vi "try.vi"() -> ()   [LabVIEW 2015]
uses:
  <vilib>/addons/_JKI.lib/REST Client/classes/REST Client/REST Client.lvclass
  <vilib>/httpClient/LabVIEWHTTPClient.lvlib
  <vilib>/httpClient/MultipartData.ctl
  <vilib>/addons/_JKI.lib/REST Client/classes/REST Client/HTTP Header.ctl
panel:
  out "error out":errorcluster
  out "Status Code 2":u16
  out "headers":string
  out "body":string
  in  "url":string
  out "error out 3":errorcluster
  in  "Same Params?":bool
  out "Status String":string
  out "Response body posting":string
  out "error out  2":errorcluster
  in  "Post Path":string="/v1/document_revisions/external/0b9ed9ad-4393-4a37-838e-578edaaebe9e"
  in  "Default Headers ([JSON]) 2":T1[](array[typedef])=[{"header"="Content-Type", "value"="application/json"}]
  in  "Base URL Posting":string="https://api.dev.enlil.io/api"
  out "Local Cluster":T2
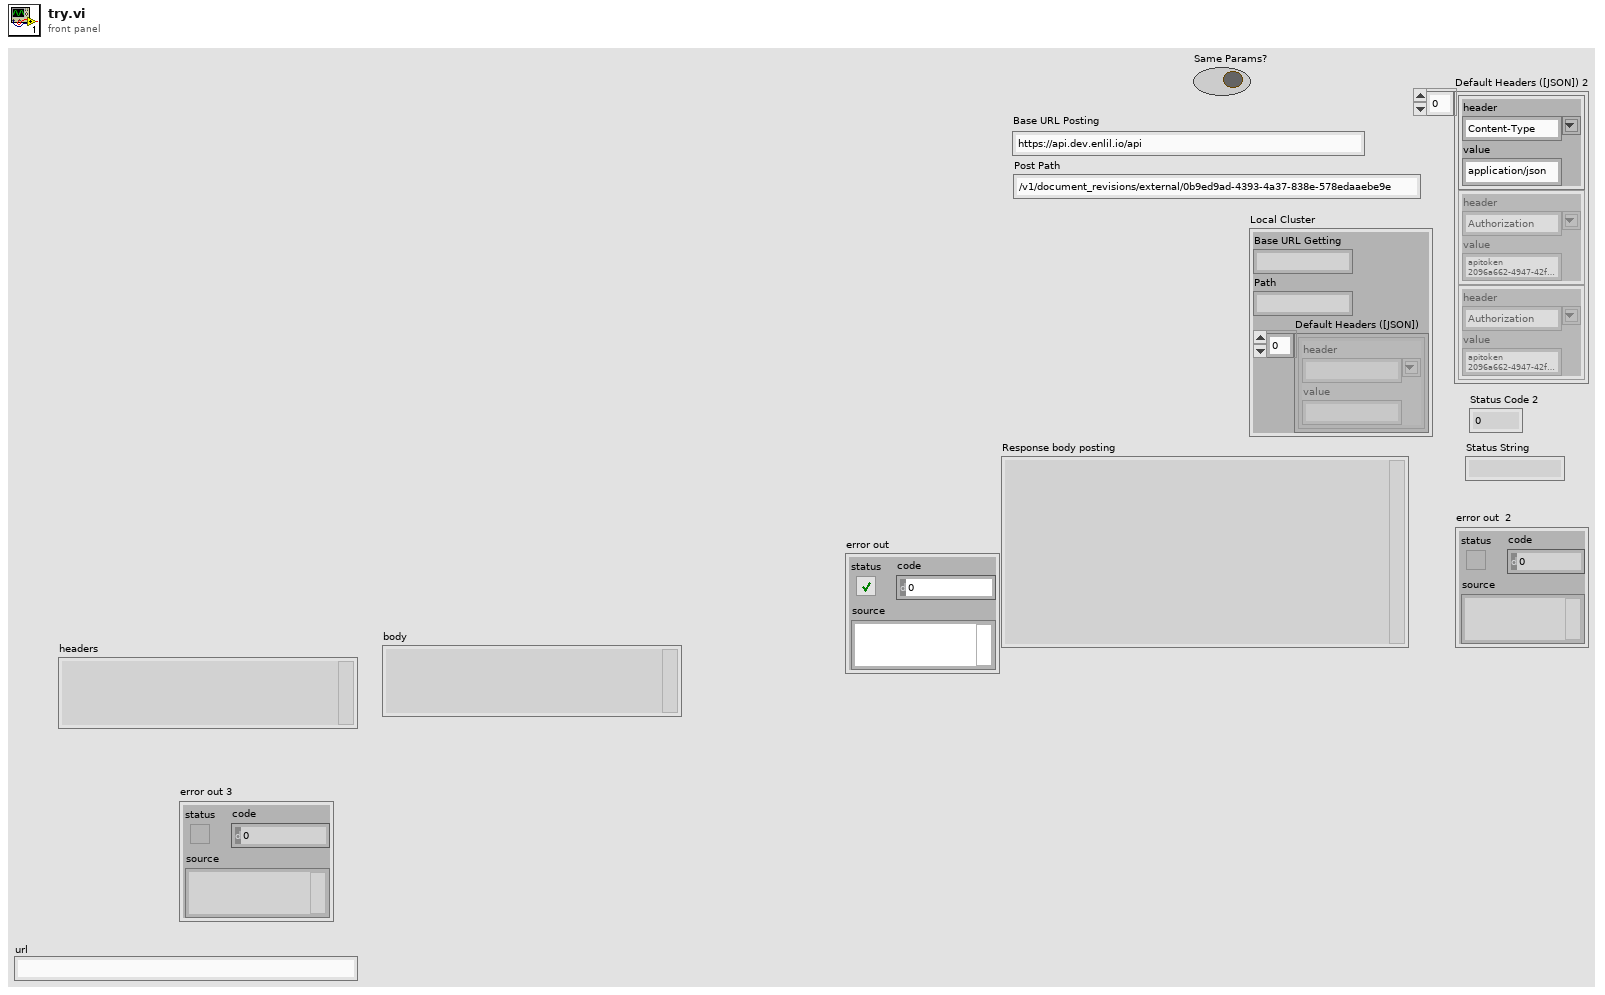
[diagram p1: front panel]
types:
  T1 = typedef "REST Client.lvlib/REST Client.lvclass/HTTP Header.ctl" = cluster{"header":string, "value":string}
  T2 = cluster{"Base URL Getting":string, "Path":string, "Default Headers ([JSON])":T1[]}
  T3 = typedef "LabVIEWHTTPClient.lvlib/MultipartData.ctl" = cluster{"Name":string, "Value":string, "File":path, "Filename":string, "MIME type":string}
  T4 = typedef "LabVIEWHTTPClient.lvlib/ClientHandle.ctl" = refnum<k1>
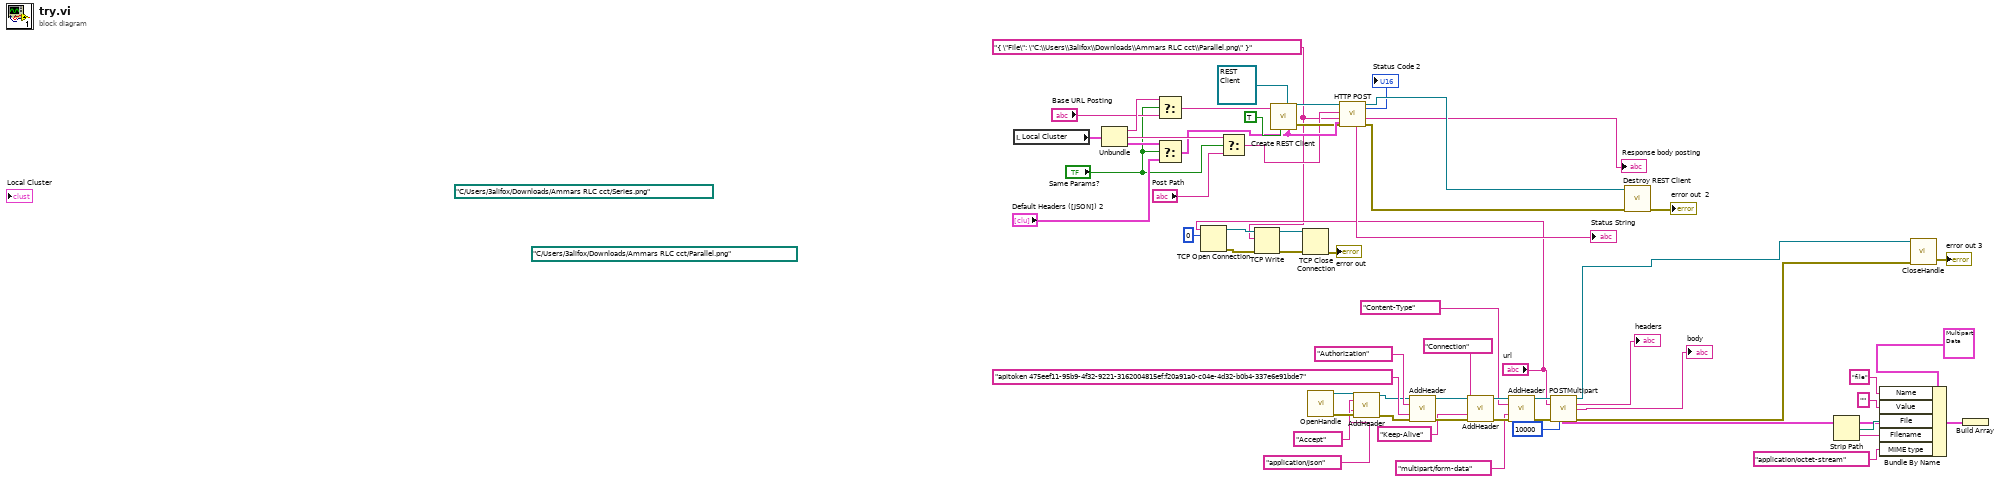
[diagram p0: block diagram]
diagram:
  (unwired) path "C:/Users/3alifox/Downloads/Ammars RLC cct/Series.png" ("Path")
  (unwired) path "C:/Users/3alifox/Downloads/Ammars RLC cct/Parallel.png" ("path to PNG file")
  w5 = "{ \"File\": \"C:\\Users\\3alifox\\Downloads\\Ammars RLC cct\\Parallel.png\" }" ("Request body")
  n1 = local read "Local Cluster"() -> (w58:T2)
  n2 = Unbundle(w58) -> ("Base URL Getting"=w57:string, "Path"=w52:string, "Default Headers ([JSON])"=w54:T1[])
  n3 = Select(t=w57, s="Same Params?", f="Base URL Posting") -> (s? t:f=w55:string)
  n4 = Select(t=w54, s="Same Params?", f="Default Headers ([JSON]) 2") -> (s? t:f=w46:T1[])
  n5 = TCP Open Connection(address="url", remote port or service name=u16 0) -> (connection ID=w8:refnum<k5>, error out=w11:errorcluster)  [unwired: 3 in]
  n6 = Select(t=w52, s="Same Params?", f="Post Path") -> (s? t:f=w43:string)
  n7 = TCP Write(connection ID=w8, data in=w5, error in (no error)=w11) -> (connection ID out=w9:refnum<k5>, error out=w10:errorcluster)  [unwired: 1 in, 1 out]
  n8 = call <vilib>:"Create REST Client.vi"("Default Headers ([JSON])"=w46, "REST Client in"=refnum<class "REST Client.lvclass"> refnum, "Verify Server(true)"=TRUE, "Base URL"=w55) -> ("error out"=w45:errorcluster, "REST Client out"=w47:refnum<class "REST Client.lvclass">)  [unwired: 6 in]
  n9 = TCP Close Connection(connection ID=w9, error in (no error)=w10) -> (error out=→"error out":errorcluster)  [unwired: 1 in, 1 out]
  n10 = call <vilib>:"OpenHandle.vi"() -> ("client handle out"=w15:T4, "error out"=w17:errorcluster)  [unwired: 14 in]
  n11 = call-dynamic "HTTP POST.vi"("request specific headers"=w46, "error in (no error)"=w45, "Request body"=w5, "Path"=w43, "REST Client in"=w47) -> ("error out"=w39:errorcluster, "Response body"=→"Response body posting":string, "REST Client out"=w44:refnum<class "REST Client.lvclass">, "Status String"=→"Status String":string, "Status Code"=→"Status Code 2":u16)  [unwired: 1 in, 1 out]
  n12 = call <vilib>:"AddHeader.vi"("client handle"=w15, "header"="Accept", "value"="application/json", "error in (no error)"=w17) -> ("client handle out"=w14:T4, "error out"=w16:errorcluster)  [unwired: 10 in]
  n13 = call <vilib>:"AddHeader.vi"("client handle"=w14, "header"="Authorization", "value"="apitoken 475eef11-95b9-4f32-9221-3162004815ef:f20a91a0-c04e-4d32-b0b4-337e6e91bde7", "error in (no error)"=w16) -> ("client handle out"=w26:T4, "error out"=w27:errorcluster)  [unwired: 10 in]
  n14 = call <vilib>:"AddHeader.vi"("client handle"=w26, "header"="Connection", "value"="Keep-Alive", "error in (no error)"=w27) -> ("client handle out"=w22:T4, "error out"=w23:errorcluster)  [unwired: 10 in]
  n15 = call <vilib>:"AddHeader.vi"("client handle"=w22, "header"="Content-Type", "value"="multipart/form-data", "error in (no error)"=w23) -> ("client handle out"=w19:T4, "error out"=w18:errorcluster)  [unwired: 10 in]
  n16 = call-dynamic "Destroy REST Client.vi"("error in (no error)"=w39, "REST Client in"=w44) -> ("error out"=→"error out  2":errorcluster)  [unwired: 9 in]
  n17 = Strip Path() -> (path=w3:path, name=w35:string)  [unwired: 1 out]
  n18 = Bundle By Name(cluster=T3 {"Name"="", "Value"="", "File"=path "", "Filename"="", "MIME type"="application/octet-stream"} ("Element"), "Name"="file", "Value"="", "File"=w3, "Filename"=w35, "MIME type"="application/octet-stream") -> (w37:T3)
  n19 = Build Array(w37) -> (w1:T3[])
  n20 = call <vilib>:"POSTMultipart.vi"("client handle"=w19, "url"="url", "data"=w1, "error in (no error)"=w18, "timeout (10000)"=10000) -> ("client handle out"=w32:T4, "headers"=→"headers":string, "body"=→"body":string, "error out"=w31:errorcluster)  [unwired: 7 in]
  n21 = call <vilib>:"CloseHandle.vi"("client handle"=w32, "error in (no error)"=w31) -> ("error out"=→"error out 3":errorcluster)  [unwired: 13 in]
